vi "WPI_CameraSend Images To PC Loop.vi"(8 "error in (no error)":errorcluster) -> ()   [LabVIEW 2016]
doc: "This VI is used to send images to the dashboard using the second enet port on the 8 slot controller. This is provided for compatibility, but is higher overhead than using the Camera MJPG approach.\n\nThis software is licensed. Open the labview\\readme\\WPI Robotics Library Open Source License.txt file for more information."
uses:
  <vilib>/Rock Robotics/Network Tables/NT Write String Array.vi
  <vilib>/Rock Robotics/Network Tables/NT Write String.vi
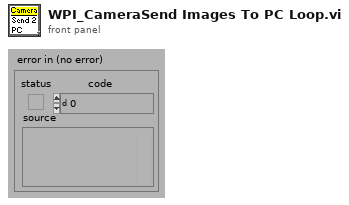
[diagram p1: front panel]
types:
  T1 = enum16{"Standard", "Buffered", "CRLF", "Immediate"}
  T2 = cluster{"token string":string, "token string 2":string}[]
  T3 = typedef "WPI_CameraDevRef.ctl" = cluster{"Camera Address":string, "CameraStatus":errorcluster}
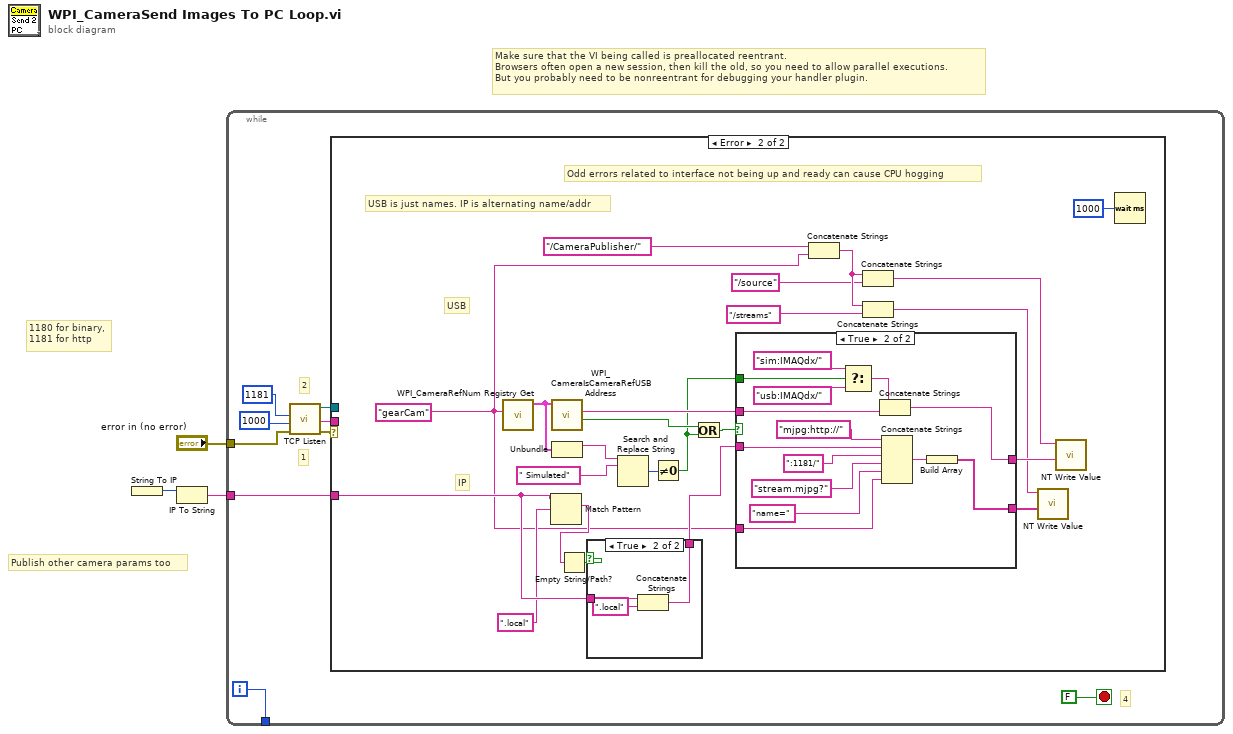
[diagram p0: block diagram]
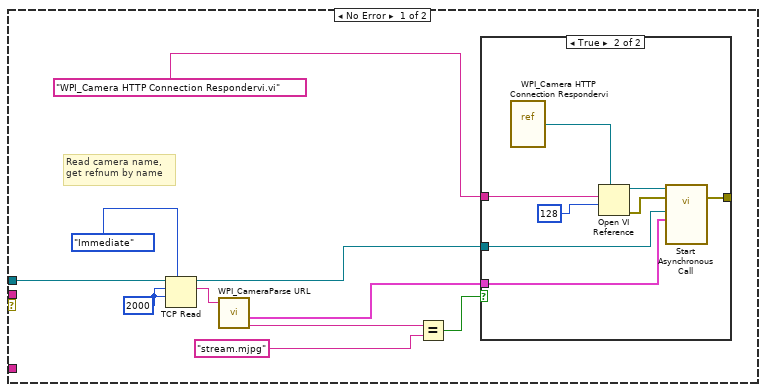
[diagram p2: hidden frame]
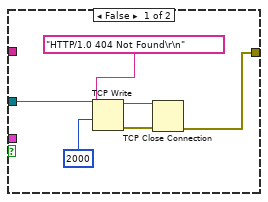
[diagram p3: hidden frame]
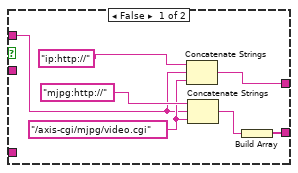
[diagram p5: hidden frame]
diagram:
  # "Make sure that the VI being called is preallocated reentrant.\nBrowsers often open a new session, then kill the old, so you need to allow parallel executions.\nBut you probably need to be nonreentrant for debugging your handler plugin."
  # "Publish other camera params too"
  # "1180 for binary,\n1181 for http"
  n1 = String To IP() -> (0:w1:u32)  [unwired: 1 in]
  n2 = IP To String(2:w1) -> (0:w2:string)  [unwired: 1 in]
  n3 = while {
    tunnel: "error in (no error)" -> [w11]
    tunnel: [w6] -> _
    tunnel: w2 -> [w4]
    i -> [w6]
    stop <- FALSE ("status") stop-if-true
    # "4"
    # "1"
    # "2"
    n4 = call <vilib>:"TCP Listen.vi"("error in (no error)"=w11, "timeout ms (wait forever: -1)"=u16 1000 ("port"), "port"=u16 1181) -> ("error out"=w8:errorcluster, "remote address"=w12:string, "connection ID"=w10:refnum<k5>)  [unwired: 1 in, 5 out]
    n5 = case shown="Error" w8 {
      tunnel: w12 -> [_ _]
      tunnel: w10 -> [w19 _]
      tunnel: w4 -> [_ w58]
      frame No Error {
        w20 = 2000
        # "Read camera name,\nget refnum by name"
        n6 = TCP Read(connection ID=w19, bytes to read=w20, 7:T1."Immediate" ("mode (standard)"), 9:w20) -> (connection ID out=w18:refnum<k5>, data out=w13:string)  [unwired: 1 in, 1 out]
        n7 = call <vilib>:"WPI_CameraParse URL.vi"("URL"=w13) -> ("cgi string"=w15:string, "parameters"=w14:T2)  [unwired: 7 in, 2 out]
        n8 = Equal?(x=w15, y="stream.mjpg") -> (x = y?=w17:bool)
        n9 = case shown="True" w17 {
          tunnel: "WPI_Camera HTTP Connection Respondervi.vi" -> [_ w36]
          tunnel: w18 -> [w28 w32]
          tunnel: [w23 w30] -> _
          tunnel: w14 -> [_ w29]
          frame False {
            n10 = TCP Write(connection ID=w28, data in="HTTP/1.0 404 Not Found\r\n" ("regular expression"), 9:2000) -> (connection ID out=w27:refnum<k5>, error out=w24:errorcluster)  [unwired: 1 in, 1 out]
            n11 = TCP Close Connection(connection ID=w27, error in (no error)=w24) -> (error out=w23:errorcluster)  [unwired: 2 out]
          }
          frame True {
            n12 = vi-ref <vilib>:"WPI_Camera HTTP Connection Respondervi.vi"() -> (w34:refnum<vi>)
            n13 = Open VI Reference(type specifier VI Refnum (for type only)=w34, vi path=w36, options=128) -> (vi reference=w33:refnum<vi>, error out=w31:errorcluster)  [unwired: 3 in]
            n14 = call-by-ref "Start Asynchronous Call"(reference=w33, error in=w31, "parameters"=w29, "connection ID"=w32) -> (error out=w30:errorcluster)  [unwired: 10 in, 1 out]
          }
        }
      }
      frame Error {
        w37 = "gearCam" ("refnum name")
        # "USB is just names. IP is alternating name/addr"
        # "IP"
        # "USB"
        # "Odd errors related to interface not being up and ready can cause CPU hogging"
        n15 = call <vilib>:"WPI_CameraRefNum Registry Get.vi"("refnum name"=w37) -> ("CameraDevRef"=w47:T3)  [unwired: 9 in, 1 out]
        n16 = Match Pattern(string=w58, regular expression=".local") -> (match substring=w38:string)  [unwired: 1 in, 3 out]
        n17 = call <vilib>:"WPI_CameraIsCameraRefUSBAddress.vi"("CameraDevRef"=w47) -> ("USB?"=w44:bool, "Camera Address Out"=w49:string)  [unwired: 7 in, 2 out]
        n18 = Unbundle(w47) -> ("Camera Address"=w46:string)  [unwired: 1 out]
        n19 = Empty String/Path?(string/path=w38) -> (empty?=w41:bool)
        n20 = case shown="True" w41 {
          tunnel: w58 -> [w60 w63]
          tunnel: [w60 w61] -> w40
          frame False {
          }
          frame True {
            n21 = Concatenate Strings(w63, ".local" ("string")) -> (w61:string)
          }
        }
        n22 = Search and Replace String(input string=w46, search string=" Simulated") -> (number of replacements=w45:i32)  [unwired: 6 in, 3 out]
        n23 = Not Equal To 0?(x=w45) -> (x != 0?=w42:bool)
        n24 = Or(x=w44, y=w42) -> (x .or. y?=w43:bool)
        n25 = case shown="True" w43 {
          tunnel: w49 -> [w66 w76]
          tunnel: w40 -> [_ w83]
          tunnel: w37 -> [_ w79]
          tunnel: [w64 w75] -> w57
          tunnel: [w68 w77] -> w50
          tunnel: w42 -> [_ w74]
          frame False {
            w67 = "/axis-cgi/mjpg/video.cgi"
            n26 = Concatenate Strings("ip:http://", w66, w67) -> (w64:string)
            n27 = Concatenate Strings("mjpg:http://", w66, w67) -> (w69:string)
            n28 = Build Array(w69) -> (w68:string[])
          }
          frame True {
            n29 = Select(t="sim:IMAQdx/", s=w74, f="usb:IMAQdx/") -> (s? t:f=w71:string)
            n30 = Concatenate Strings(w71, w76) -> (w75:string)
            n31 = Concatenate Strings("mjpg:http://", w83, ":1181/", "stream.mjpg?", "name=", w79) -> (w78:string)
            n32 = Build Array(w78) -> (w77:string[])
          }
        }
        n33 = Concatenate Strings("/CameraPublisher/", w37) -> (w54:string)
        n34 = Concatenate Strings(w54, "/source") -> (w51:string)
        n35 = Concatenate Strings(w54, "/streams") -> (w52:string)
        n36 = call-poly <vilib>:"NT Write Value.vi"("String Array"=w50, "Name"=w52) -> ()  [unwired: 9 in, 1 out]
        n37 = call-poly <vilib>:"NT Write Value.vi"("String"=w57, "Name"=w51) -> ()  [unwired: 9 in, 1 out]
        n38 = Wait (ms)(milliseconds to wait=u32 1000) -> ()  [unwired: 1 out]
      }
    }
  }
